vi "Create Box Plot.vi"(5 "Width per Box Plot":dbl=10.0 format="%.2f", 11 "Raw Box Plot Data":cluster{"Samples":dbl[]}[](array[cluster])) -> (0 "min":dbl, 1 "max":dbl, 2 "Number of Plots":i32, 3 "Box Plots":cluster{dbl[], dbl[]}[](array[cluster]))   [LabVIEW 2022 SP3, in "Box Plots.lvlib"]
uses:
  Box Plots.lvlib
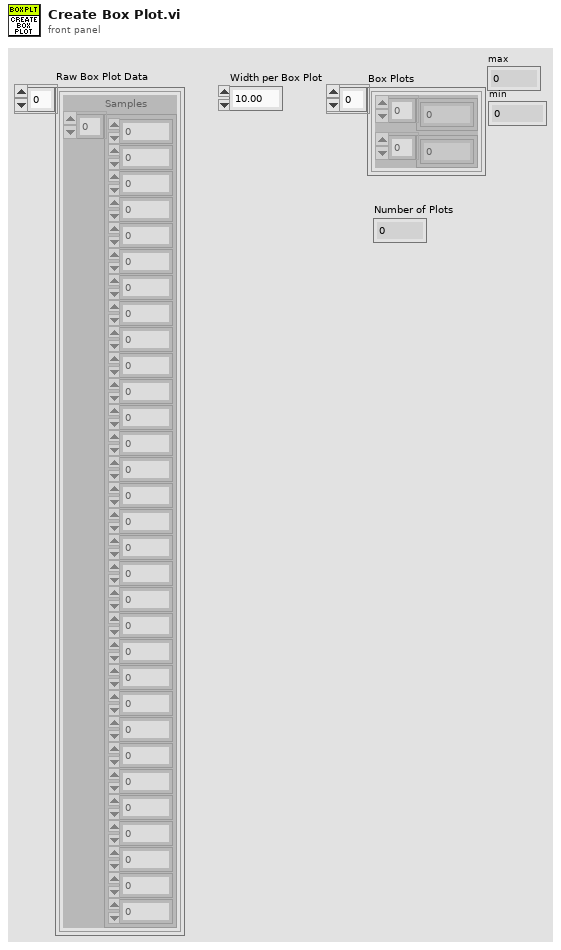
[diagram p1: front panel]
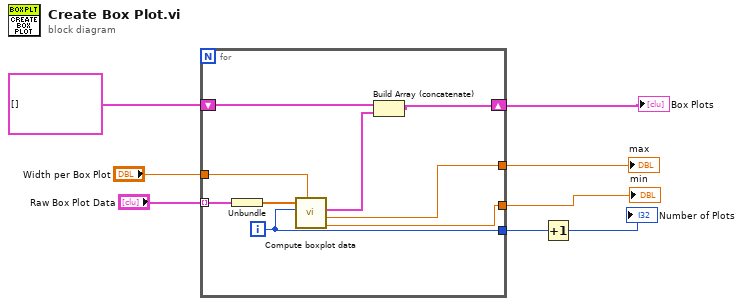
[diagram p0: block diagram]
diagram:
  n1 = for {
    tunnel: "Raw Box Plot Data" -> [w17] mode=indexing
    tunnel: [w15] -> w6
    tunnel: "Width per Box Plot" -> [w14]
    shift-right: [w13] -> w7
    shift-left: cluster{dbl[], dbl[]}[] [] ("array") -> [w11]
    tunnel: [w10] -> w2
    tunnel: [w9] -> w1
    i -> [w15]
    n2 = Unbundle(w17) -> ("Samples"=w16:dbl[])
    n3 = call "Compute boxplot data.vi"("Box Width"=w14, "Plot #"=w15, "Raw Data"=w16) -> ("min"=w9:dbl, "max"=w10:dbl, "XY Graph"=w12:cluster{dbl[], dbl[]}[])  [unwired: 2 in, 3 out]
    n4 = Build Array (concatenate)(w11, w12) -> (w13:cluster{dbl[], dbl[]}[])
  }
  "Box Plots" <- w7
  "max" <- w2
  "min" <- w1
  n5 = Increment(x=w6) -> (x+1=→"Number of Plots":i32)
